vi "Untitled 1.vi"   [LabVIEW 2020]
uses:
  Classes/Workspace/Component/Component Tray.lvclass
  Projects/Sensor Dispense.lvclass
  Classes/Controller/Controller.lvclass
types:
  T1 = typedef "Controller.lvclass/Controllers.ctl" = cluster{"I-O.lvclass":refnum<class "I-O.lvclass">, "Dispenser.lvclass":refnum<class "Dispenser.lvclass">, "Gantry":refnum<k24>}
  T2 = typedef "Fixture.lvclass/Workspace.ctl" = cluster{"XYZTheta":dbl[], "Workspace Valve":i32, "Workspace Sensor":i32}
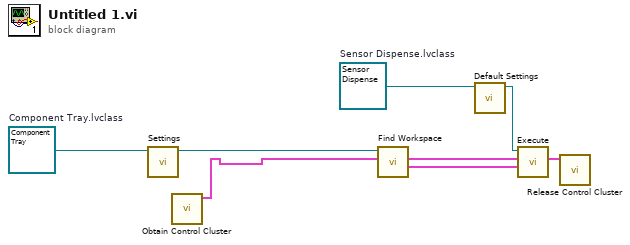
[diagram p0: block diagram]
diagram:
  w7 = refnum<class "Sensor Dispense.lvclass"> refnum  # Sensor Dispense.lvclass
  w8 = refnum<class "Component Tray.lvclass"> refnum  # Component Tray.lvclass
  n1 = call-dynamic "Settings.vi"("Component in"=w8) -> ("Component out"=w1:refnum<class "Component Tray.lvclass">)  [unwired: 9 in, 1 out]
  n2 = call "Obtain Control Cluster.vi"() -> ("Control Out"=w2:T1)  [unwired: 11 in]
  n3 = call-dynamic "Find Workspace.vi"("Control In"=w2, "Component.lvclass"=w1) -> ("Workspace"=w5:T2, "Control Out"=w4:T1)  [unwired: 6 in, 2 out]
  n4 = call-dynamic "Default Settings.vi"("Sensor Dispense in"=w7) -> ("Sensor Dispense out"=w6:refnum<class "Sensor Dispense.lvclass">)  [unwired: 9 in, 1 out]
  n5 = call-dynamic "Execute.vi"("Workspace"=w5, "Control In"=w4, "Dispense in"=w6) -> ("Control Out"=w3:T1)  [unwired: 6 in, 2 out]
  n6 = call "Release Control Cluster.vi"("output cluster"=w3) -> ()  [unwired: 11 in]
